vi "Control ITC Sweep -- aggregate state.vi"(8 "error in":errorcluster, 10 "more state":T2={"time(min)"=0.0, "T (ITC )"=295.7, "T (ITC, set)"=295.7, "heater"=3.3, "gas"=99.9, "T (ITC)  - T (ITC, set)"=-0.0036623472822157055, "T (LTC)  - T (ITC, set)"=-0.029662347282226165, "heater slope"=-0.026390225842280686, "LTC slope"=0.11130455386895922, "hetaer running average"=3.211444650129601, "T (LTC)"=295.674, "T (LTC) running average"=295.6704744761195}, 11 "more state -- aggregate in":T1={"time(min)"=array[7200 elements], "T (ITC )"=array[7200 elements], "T (ITC, set)"=array[7200 elements], "T (LTC)"=array[7200 elements], "heater"=array[7200 elements], "gas"=array[7200 elements], "T (ITC)  - T (ITC, set)"=array[7200 elements], "T (LTC)  - T (ITC, set)"=array[7200 elements], "heater slope"=array[7200 elements], "LTC slope"=array[7200 elements], "hetaer running average"=array[7200 elements], "T (LTC) running average"=array[7200 elements]}) -> (0 "error out":errorcluster, 3 "more state -- aggregate out":T1)   [LabVIEW 2010]
uses:
  collect.ctl
  collect - input.ctl
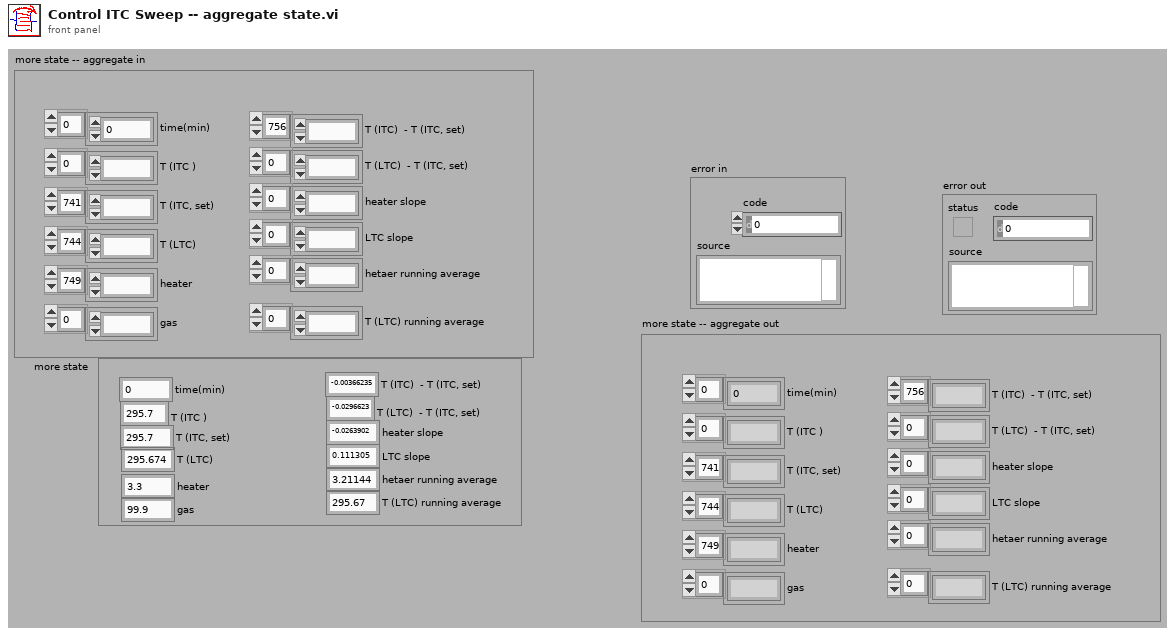
[diagram p1: front panel]
types:
  T1 = typedef "collect.ctl" = cluster{"time(min)":dbl[], "T (ITC )":dbl[], "T (ITC, set)":dbl[], "T (LTC)":dbl[], "heater":dbl[], "gas":dbl[], "T (ITC)  - T (ITC, set)":dbl[], "T (LTC)  - T (ITC, set)":dbl[], "heater slope":dbl[], "LTC slope":dbl[], "hetaer running average":dbl[], "T (LTC) running average":dbl[]}
  T2 = typedef "collect - input.ctl" = cluster{"time(min)":dbl, "T (ITC )":dbl, "T (ITC, set)":dbl, "heater":dbl, "gas":dbl, "T (ITC)  - T (ITC, set)":dbl, "T (LTC)  - T (ITC, set)":dbl, "heater slope":dbl, "LTC slope":dbl, "hetaer running average":dbl, "T (LTC)":dbl, "T (LTC) running average":dbl}
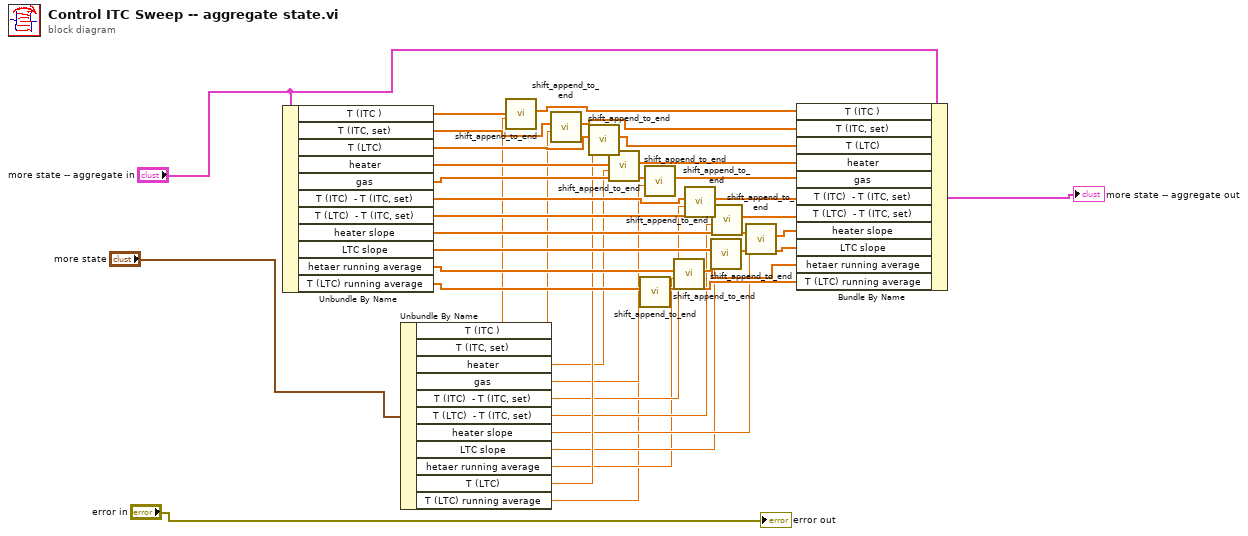
[diagram p0: block diagram]
diagram:
  n1 = Unbundle By Name("more state -- aggregate in") -> ("T (ITC )"=w19:dbl[], "T (ITC, set)"=w17:dbl[], "T (LTC)"=w36:dbl[], "heater"=w35:dbl[], "gas"=w32:dbl[], "T (ITC)  - T (ITC, set)"=w25:dbl[], "T (LTC)  - T (ITC, set)"=w20:dbl[], "heater slope"=w21:dbl[], "LTC slope"=w22:dbl[], "hetaer running average"=w23:dbl[], "T (LTC) running average"=w24:dbl[])
  n2 = Unbundle By Name("more state") -> ("T (ITC )"=w15:dbl, "T (ITC, set)"=w14:dbl, "heater"=w12:dbl, "gas"=w11:dbl, "T (ITC)  - T (ITC, set)"=w10:dbl, "T (LTC)  - T (ITC, set)"=w9:dbl, "heater slope"=w8:dbl, "LTC slope"=w7:dbl, "hetaer running average"=w6:dbl, "T (LTC)"=w13:dbl, "T (LTC) running average"=w5:dbl)
  n3 = call "shift_append_to_end.vi"("new element"=w15, "input array"=w19) -> ("output array"=w18:dbl[])  [unwired: 9 in]
  n4 = call "shift_append_to_end.vi"("new element"=w14, "input array"=w17) -> ("output array"=w16:dbl[])  [unwired: 9 in]
  n5 = call "shift_append_to_end.vi"("new element"=w13, "input array"=w36) -> ("output array"=w37:dbl[])  [unwired: 9 in]
  n6 = call "shift_append_to_end.vi"("new element"=w12, "input array"=w35) -> ("output array"=w34:dbl[])  [unwired: 9 in]
  n7 = call "shift_append_to_end.vi"("new element"=w5, "input array"=w24) -> ("output array"=w26:dbl[])  [unwired: 9 in]
  n8 = call "shift_append_to_end.vi"("new element"=w11, "input array"=w32) -> ("output array"=w33:dbl[])  [unwired: 9 in]
  n9 = call "shift_append_to_end.vi"("new element"=w6, "input array"=w23) -> ("output array"=w27:dbl[])  [unwired: 9 in]
  n10 = call "shift_append_to_end.vi"("new element"=w10, "input array"=w25) -> ("output array"=w31:dbl[])  [unwired: 9 in]
  n11 = call "shift_append_to_end.vi"("new element"=w7, "input array"=w22) -> ("output array"=w28:dbl[])  [unwired: 9 in]
  n12 = call "shift_append_to_end.vi"("new element"=w9, "input array"=w20) -> ("output array"=w30:dbl[])  [unwired: 9 in]
  n13 = call "shift_append_to_end.vi"("new element"=w8, "input array"=w21) -> ("output array"=w29:dbl[])  [unwired: 9 in]
  n14 = Bundle By Name(cluster="more state -- aggregate in", "T (ITC )"=w18, "T (ITC, set)"=w16, "T (LTC)"=w37, "heater"=w34, "gas"=w33, "T (ITC)  - T (ITC, set)"=w31, "T (LTC)  - T (ITC, set)"=w30, "heater slope"=w29, "LTC slope"=w28, "hetaer running average"=w27, "T (LTC) running average"=w26) -> (→"more state -- aggregate out":T1)
  "error out" <- "error in"
